vi "Set View Position.vi"(8 "error in (no error)":errorcluster, 10 "Position":T1, 11 "TabControlRef in":refnum<vi>) -> (0 "error out":errorcluster, 3 "TabControlRef out":refnum<vi>)   [LabVIEW 2020, in "MDI ViewManager.lvlib"]
uses:
  MDI ViewManager.lvlib
  <vilib>/Utility/miscctls.llb/LVPositionTypeDef.ctl
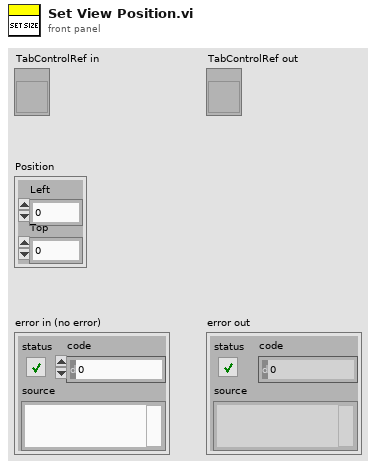
[diagram p1: front panel]
types:
  T1 = typedef "LVPositionTypeDef.ctl" = cluster{"Left":i32, "Top":i32}
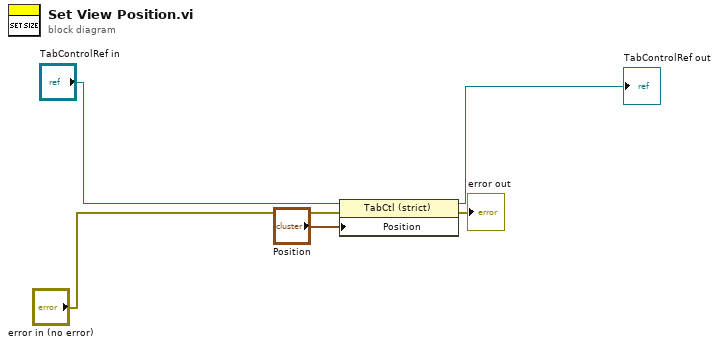
[diagram p0: block diagram]
diagram:
  n1 = property class="TabCtl (strict)"(reference="TabControlRef in", error in="error in (no error)", "Position"="Position") -> (reference out=→"TabControlRef out":refnum<vi>, error out=→"error out":errorcluster)
